vi "TMC INIT.vi"   [LabVIEW 2010]
uses:
  TPS Global.vi
  <vilib>/Utility/config.llb/Read Key (I32).vi
  TMC Global.vi
  <vilib>/Utility/config.llb/Read Key (String).vi
  <vilib>/Utility/config.llb/NI_LVConfig.lvlib
types:
  T1 = typedef "NI_LVConfig.lvlib/Config Data RefNum.ctl" = refnum<k1>
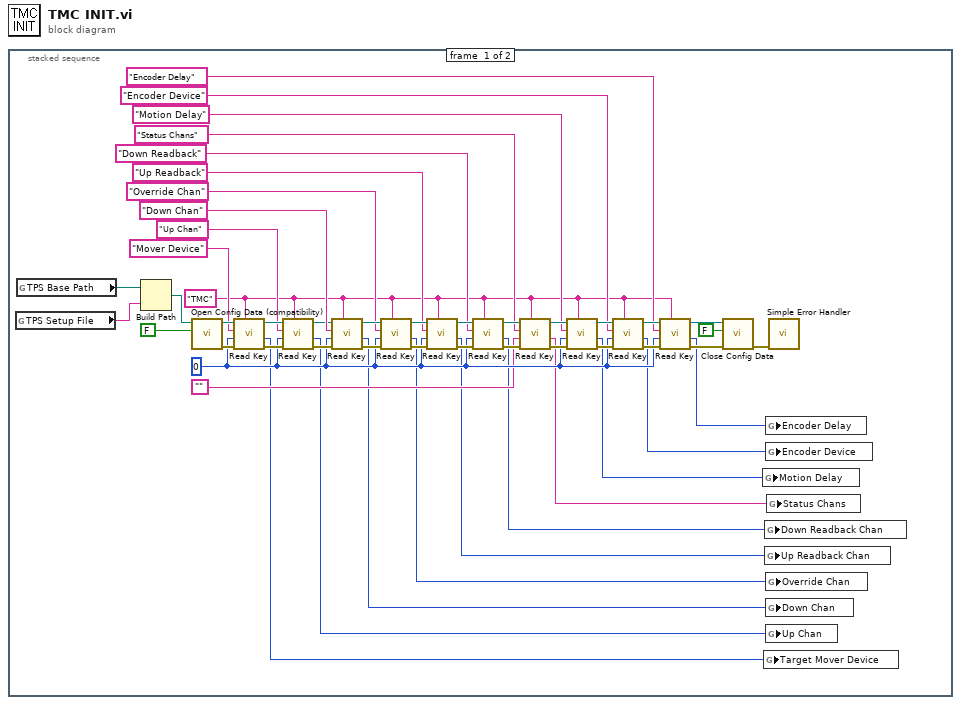
[diagram p0: block diagram]
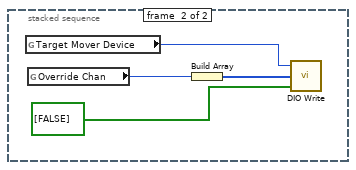
[diagram p2: hidden frame]
diagram:
  n1 = stacked-sequence {
    frame #0 {
      w14 = 0
      w2 = "TMC" ("section")
      n2 = global read "TPS Global.vi" "TPS Setup File"() -> (w38:string)
      n3 = global read "TPS Global.vi" "TPS Base Path"() -> (w51:path)
      n4 = Build Path(base path=w51, name or relative path=w38) -> (appended path=w43:path)
      n5 = call <vilib>:"Open Config Data (compatibility).vi"("create file if necessary (T)"=FALSE ("create file if necessary? (T)"), "configuration file path"=w43) -> ("error out"=w41:errorcluster, "refnum"=w40:T1)  [unwired: 7 in, 1 out]
      n6 = call-poly <vilib>:"Read Key.vi"("section"=w2, "error in (no error)"=w41, "default value"=w14, "key"="Mover Device", "refnum"=w40) -> ("error out"=w45:errorcluster, "value"=w3:i32, "refnum out"=w46:T1)  [unwired: 3 in, 1 out]
      n7 = call-poly <vilib>:"Read Key.vi"("section"=w2, "error in (no error)"=w45, "default value"=w14, "key"="Up Chan", "refnum"=w46) -> ("error out"=w48:errorcluster, "value"=w4:i32, "refnum out"=w49:T1)  [unwired: 3 in, 1 out]
      n8 = call-poly <vilib>:"Read Key.vi"("section"=w2, "error in (no error)"=w48, "default value"=w14, "key"="Down Chan", "refnum"=w49) -> ("error out"=w23:errorcluster, "value"=w5:i32, "refnum out"=w22:T1)  [unwired: 3 in, 1 out]
      n9 = call-poly <vilib>:"Read Key.vi"("section"=w2, "error in (no error)"=w23, "default value"=w14, "key"="Override Chan", "refnum"=w22) -> ("error out"=w37:errorcluster, "value"=w6:i32, "refnum out"=w36:T1)  [unwired: 3 in, 1 out]
      n10 = call-poly <vilib>:"Read Key.vi"("section"=w2, "error in (no error)"=w37, "default value"=w14, "key"="Up Readback", "refnum"=w36) -> ("error out"=w35:errorcluster, "value"=w7:i32, "refnum out"=w34:T1)  [unwired: 3 in, 1 out]
      n11 = call-poly <vilib>:"Read Key.vi"("section"=w2, "error in (no error)"=w35, "default value"=w14, "key"="Down Readback", "refnum"=w34) -> ("error out"=w33:errorcluster, "value"=w8:i32, "refnum out"=w32:T1)  [unwired: 3 in, 1 out]
      n12 = call-poly <vilib>:"Read Key.vi"("section"=w2, "error in (no error)"=w33, "default value"="", "key"="Status Chans", "refnum"=w32) -> ("error out"=w31:errorcluster, "value"=w12:string, "refnum out"=w30:T1)  [unwired: 3 in, 1 out]
      n13 = call-poly <vilib>:"Read Key.vi"("section"=w2, "error in (no error)"=w31, "default value"=w14, "key"="Motion Delay", "refnum"=w30) -> ("error out"=w29:errorcluster, "value"=w9:i32, "refnum out"=w28:T1)  [unwired: 3 in, 1 out]
      n14 = call-poly <vilib>:"Read Key.vi"("section"=w2, "error in (no error)"=w29, "default value"=w14, "key"="Encoder Device", "refnum"=w28) -> ("error out"=w27:errorcluster, "value"=w10:i32, "refnum out"=w26:T1)  [unwired: 3 in, 1 out]
      n15 = call-poly <vilib>:"Read Key.vi"("section"=w2, "error in (no error)"=w27, "default value"=w14, "key"="Encoder Delay", "refnum"=w26) -> ("error out"=w25:errorcluster, "value"=w11:i32, "refnum out"=w24:T1)  [unwired: 3 in, 1 out]
      n16 = call <vilib>:"Close Config Data.vi"("error in (no error)"=w25, "write file if changed (T)"=FALSE, "refnum"=w24) -> ("error out"=w47:errorcluster)  [unwired: 7 in, 1 out]
      n17 = global write "TMC Global.vi" "Motion Delay"(w9) -> ()
      n18 = global write "TMC Global.vi" "Target Mover Device"(w3) -> ()
      n19 = global write "TMC Global.vi" "Down Readback Chan"(w8) -> ()
      n20 = global write "TMC Global.vi" "Up Readback Chan"(w7) -> ()
      n21 = global write "TMC Global.vi" "Encoder Delay"(w11) -> ()
      n22 = global write "TMC Global.vi" "Encoder Device"(w10) -> ()
      n23 = global write "TMC Global.vi" "Override Chan"(w6) -> ()
      n24 = global write "TMC Global.vi" "Down Chan"(w5) -> ()
      n25 = global write "TMC Global.vi" "Up Chan"(w4) -> ()
      n26 = global write "TMC Global.vi" "Status Chans"(w12) -> ()
      n27 = call <vilib>:"Simple Error Handler.vi"("error in (no error)"=w47) -> ()  [unwired: 4 in, 5 out]
    }
    frame #1 {
      n28 = global read "TMC Global.vi" "Target Mover Device"() -> (w54:i32)
      n29 = global read "TMC Global.vi" "Override Chan"() -> (w52:i32)
      n30 = Build Array(w52) -> (w53:i32[])
      n31 = call "DIO Write.vi"("Data"=bool[] [FALSE], "Channels"=w53, "device"=w54) -> ()  [unwired: 1 out]
    }
  }
